vi "Calculate_OUR.vi"(0 "Model_Predictor in":refnum<class "Model_Predictor.lvclass">, 5 "Modify model OUR":bool, 7 "OUR calc period":dbl=60.0 format="%#_13g", 9 "CV":bool, 11 "error in (no error)":errorcluster) -> (4 "Model_Predictor out":refnum<class "Model_Predictor.lvclass">, 8 "OUR":dbl format="%#_13g", 15 "error out":errorcluster)   [LabVIEW 2021, in "MBPOnOff_Controller.lvlib" / "Model_Predictor.lvclass"]
uses:
  Model_Predictor.lvclass
  Model_Predictor.lvclass/Model_Predictor.ctl
  <vilib>/Analysis/NI_AALPro.lvlib
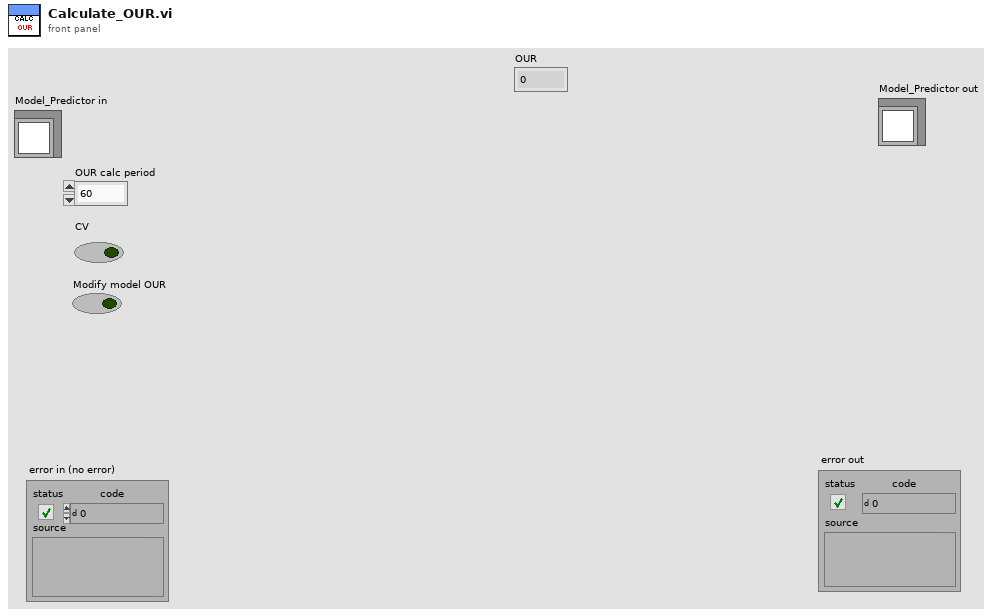
[diagram p1: front panel]
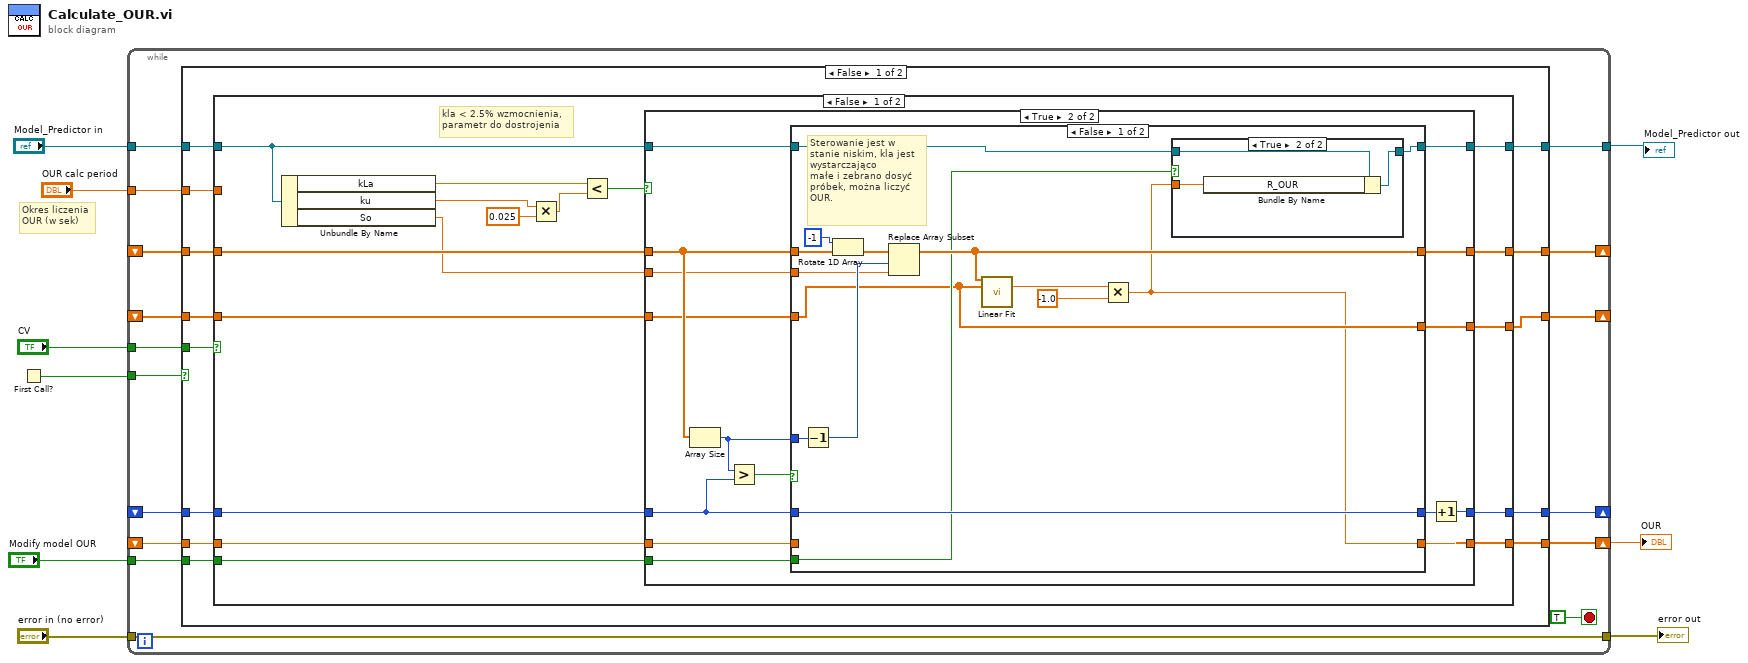
[diagram p0: block diagram]
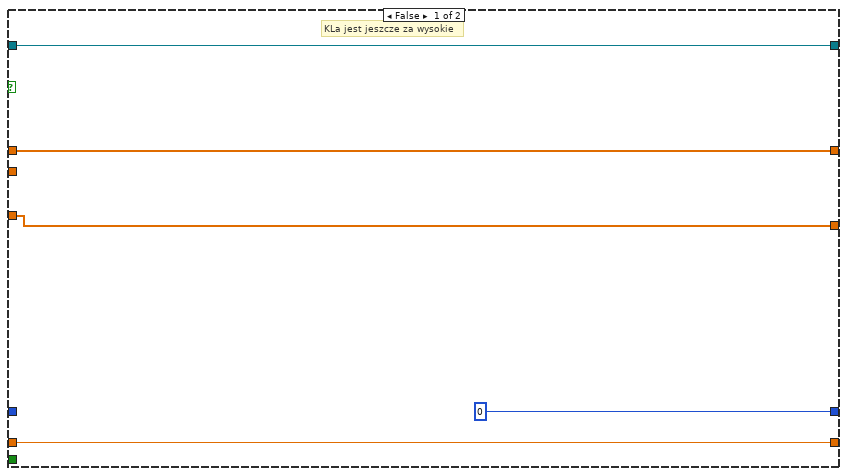
[diagram p2: hidden frame]
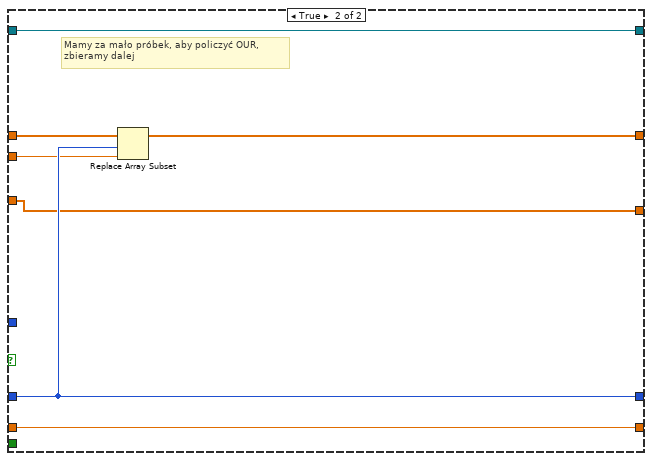
[diagram p4: hidden frame]
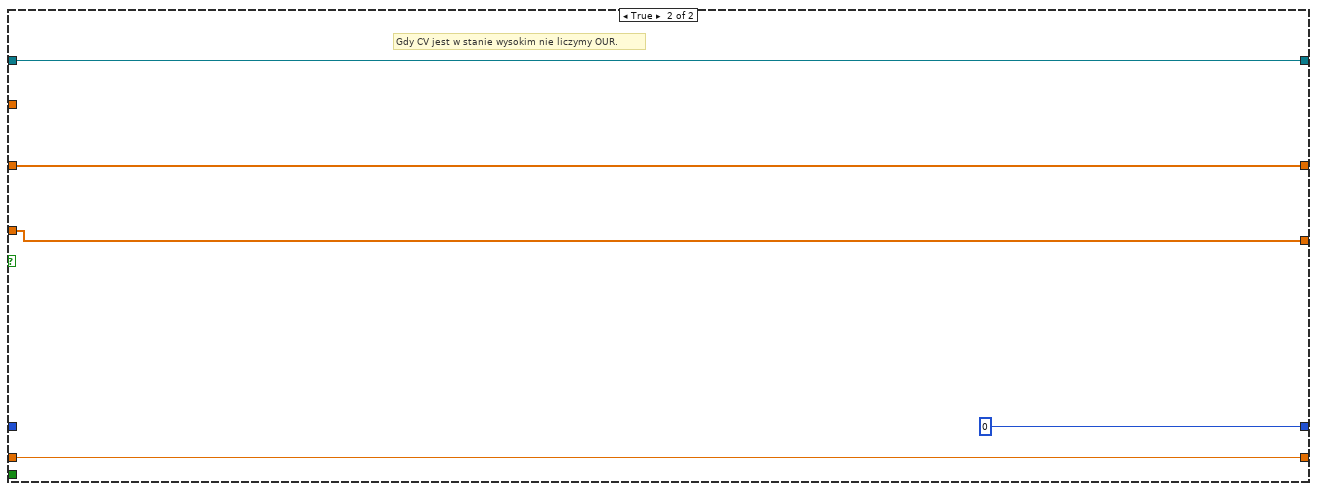
[diagram p5: hidden frame]
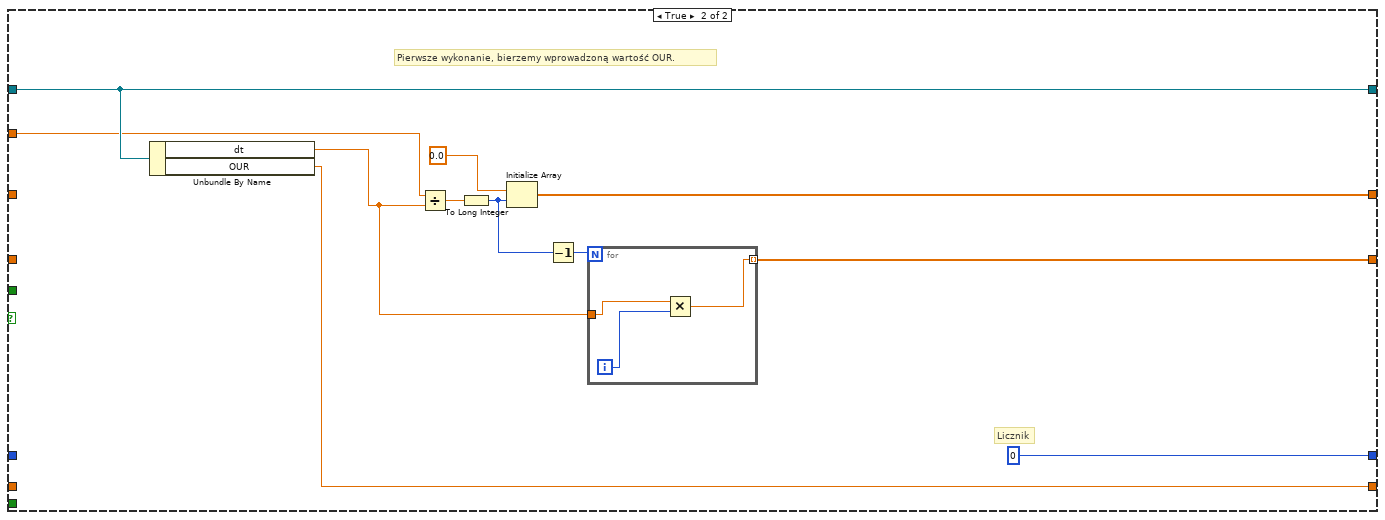
[diagram p6: hidden frame]
diagram:
  # "Okres liczenia\nOUR (w sek)"
  n1 = First Call?() -> (First Call?: T/F=w4:bool)
  n2 = while {
    tunnel: "Model_Predictor in" -> [w23]
    tunnel: [w22] -> w8
    tunnel: "CV" -> [w19]
    tunnel: [w25] -> w6
    tunnel: "error in (no error)" -> [w25]
    tunnel: w4 -> [w24]
    shift-right: [w21] -> w3
    shift-left: _ -> [w18]
    shift-right: [w17] -> _
    shift-left: _ -> [w16]
    shift-right: [w15] -> _
    shift-left: _ -> [w14]
    tunnel: "OUR calc period" -> [w13]
    shift-right: [w12] -> _
    shift-left: _ -> [w11]
    tunnel: "Modify model OUR" -> [w10]
    stop <- TRUE stop-if-true
    n3 = case shown="False" w24 {
      tunnel: w23 -> [w37 w117]
      tunnel: [w36 w117] -> w22
      tunnel: [w34 w116] -> w21
      tunnel: w19 -> [w38 _]
      tunnel: w18 -> [w35 _]
      tunnel: [w30 w113] -> w17
      tunnel: w16 -> [w31 _]
      tunnel: [w32 0] -> w15
      tunnel: w14 -> [w33 _]
      tunnel: w13 -> [w29 w111]
      tunnel: [w26 w108] -> w12
      tunnel: w11 -> [w28 _]
      tunnel: w10 -> [w27 _]
      frame False {
        n4 = case shown="False" w38 {
          tunnel: w37 -> [w50 w106]
          tunnel: [w42 w106] -> w36
          tunnel: w35 -> [w49 w105]
          tunnel: [w46 w105] -> w34
          tunnel: w33 -> [w47 _]
          tunnel: [w48 0] -> w32
          tunnel: w31 -> [w45 w104]
          tunnel: [w44 w104] -> w30
          tunnel: w29 -> [_ _]
          tunnel: w28 -> [w41 w102]
          tunnel: w27 -> [w40 _]
          tunnel: [w39 w102] -> w26
          frame False {
            # "kla < 2.5% wzmocnienia,\nparametr do dostrojenia"
            n5 = Unbundle By Name(w50) -> ("kLa"=w52:dbl, "ku"=w54:dbl, "So"=w43:dbl)
            n6 = Multiply(x=w54, y=0.025) -> (x*y=w53:dbl)
            n7 = Less?(x=w52, y=w53) -> (x < y?=w51:bool)
            n8 = case shown="True" w51 {
              tunnel: w50 -> [w57 w68]
              tunnel: w49 -> [w59 w64]
              tunnel: [0 w72] -> w48
              tunnel: w47 -> [_ w74]
              tunnel: [w59 w65] -> w46
              tunnel: w45 -> [w58 w71]
              tunnel: [w58 w70] -> w44
              tunnel: w43 -> [_ w69]
              tunnel: [w57 w63] -> w42
              tunnel: w41 -> [w56 w66]
              tunnel: w40 -> [_ w62]
              tunnel: [w56 w61] -> w39
              frame False {
                # "KLa jest jeszcze za wysokie"
              }
              frame True {
                n9 = Array Size(array=w71) -> (size(s)=w67:i32)
                n10 = Greater?(x=w67, y=w74) -> (0:w75:bool)
                n11 = case shown="False" w75 {
                  tunnel: w74 -> [w84 w101]
                  tunnel: [w84 w101] -> w73
                  tunnel: w71 -> [w90 w100]
                  tunnel: [w83 w99] -> w70
                  tunnel: w69 -> [w85 w98]
                  tunnel: w68 -> [w79 w96]
                  tunnel: w67 -> [w87 _]
                  tunnel: w66 -> [w77 w95]
                  tunnel: [w76 w97] -> w65
                  tunnel: w64 -> [_ w97]
                  tunnel: [w78 w96] -> w63
                  tunnel: w62 -> [w80 _]
                  tunnel: [w77 w95] -> w61
                  frame False {
                    # "Sterowanie jest w stanie niskim, kla jest wystarczająco\nmałe i zebrano dosyć próbek, można liczyć OUR."
                    n12 = Decrement(x=w87) -> (x-1=w86:i32)
                    n13 = Rotate 1D Array(1:w90, 2:-1 ("n")) -> (0:w88:dbl[])
                    n14 = Replace Array Subset(array=w88, new element=w85, index=w86) -> (w83:dbl[])
                    n15 = call <vilib>:"Linear Fit.vi"("Y"=w83, "X"=w77) -> ("slope"=w82:dbl)  [unwired: 9 in, 4 out]
                    n16 = Multiply(x=w82, y=-1.0) -> (x*y=w76:dbl)
                    n17 = case shown="True" w80 {
                      tunnel: w79 -> [w91 w94]
                      tunnel: [w91 w93] -> w78
                      tunnel: w76 -> [_ w92]
                      frame False {
                      }
                      frame True {
                        n18 = Bundle By Name(cluster=w94, "R_OUR"=w92) -> (w93:refnum<class "Model_Predictor.lvclass">)
                      }
                    }
                  }
                  frame True {
                    # "Mamy za mało próbek, aby policzyć OUR,\nzbieramy dalej"
                    n19 = Replace Array Subset(array=w100, new element=w98, index=w101) -> (w99:dbl[])
                  }
                }
                n20 = Increment(x=w73) -> (x+1=w72:i32)
              }
            }
          }
          frame True {
            # "Gdy CV jest w stanie wysokim nie liczymy OUR."
          }
        }
      }
      frame True {
        # "Licznik"
        # "Pierwsze wykonanie, bierzemy wprowadzoną wartość OUR."
        n21 = Unbundle By Name(w117) -> ("dt"=w107:dbl, "OUR"=w116:dbl)
        n22 = Divide(x=w111, y=w107) -> (x/y=w114:dbl)
        n23 = To Long Integer(number=w114) -> (32bit integer=w109:i32)
        n24 = Initialize Array(0.0 ("element"), w109) -> (w113:dbl[])
        n25 = Decrement(x=w109) -> (x-1=w110:i32)
        n26 = for {
          N: w110 -> [_]
          tunnel: [w120] -> w108 mode=indexing
          tunnel: w107 -> [w118]
          i -> [w119]
          n27 = Multiply(x=w118, y=w119) -> (x*y=w120:dbl)
        }
      }
    }
  }
  "Model_Predictor out" <- w8
  "error out" <- w6
  "OUR" <- w3
